vi "Send Plugin Command.vi"(6 "overwrite on timeout (T)":bool, 8 "error in (no error)":errorcluster, 9 "timeout in ms (0)":i32 format="%d ms", 10 "command":T1={"Command"=enum."Rx", "Parameters"={"arg1"=0, "arg2"=0}}, 11 "Plugin Interface in":refnum<class "Plugin Interface.lvclass">) -> (0 "error out":errorcluster, 3 "Plugin Interface out":refnum<class "Plugin Interface.lvclass">)   [LabVIEW 2020, in "DSF Core.lvlib" / "Plugin Interface.lvclass"]
uses:
  Plugin Interface.lvclass
  Interface.lvclass
  C:/Users/nitest/Desktop/Git/niveristand-data-sharing-framework-custom-device/Source/Core/Classes/Interface/Interface.lvclass
  C:/Users/nitest/Desktop/Git/niveristand-data-sharing-framework-custom-device/Source/Core/Classes/Interface/Plugin/Plugin Interface.lvclass
  Dispatcher/Command Timeout.vi
  DSF Core.lvlib
  Command.ctl
  Command Data.ctl
  Command Parameters.ctl
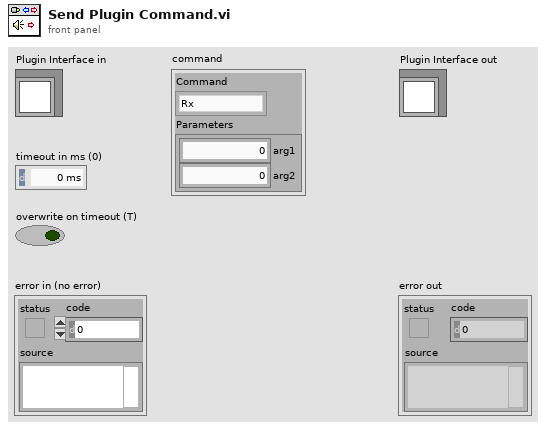
[diagram p1: front panel]
types:
  T1 = typedef "DSF Core.lvlib/Plugin Interface.lvclass/Command Data.ctl" = cluster{"Command":T2, "Parameters":T3}
  T2 = typedef "DSF Core.lvlib/Plugin Interface.lvclass/Command.ctl" = enum8{"Idle", "Start", "Set Inline Buffer", "Rx", "Tx", "Shutdown", "Error"}
  T3 = typedef "DSF Core.lvlib/Plugin Interface.lvclass/Command Parameters.ctl" = cluster{"arg1":u64, "arg2":u64}
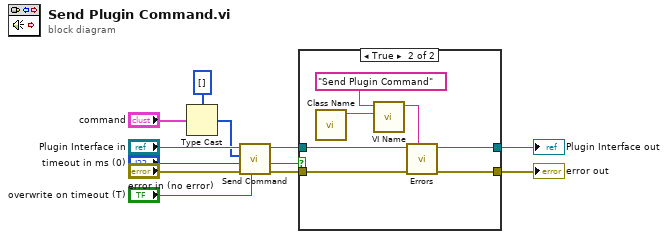
[diagram p0: block diagram]
diagram:
  n1 = Type Cast(type=u8[] [] ("element"), x="command") -> (*(type *) &x=w10:u8[])
  n2 = call "Send Command.vi"("overwrite on timeout (T)"="overwrite on timeout (T)", "error in (no error)"="error in (no error)", "timeout in ms (0)"="timeout in ms (0)", "command data"=w10, "Interface in"="Plugin Interface in") -> ("error out"=w5:errorcluster, "timed out?"=w4:bool, "Interface out"=w6:refnum<class "Plugin Interface.lvclass">)  [unwired: 3 in, 1 out]
  n3 = case shown="True" w4 {
    tunnel: w5 -> [w13 w20]
    tunnel: w6 -> [w14 w21]
    tunnel: [w14 w19] -> w3
    tunnel: [w13 w18] -> w2
    frame False {
    }
    frame True {
      n4 = call "Class Name.vi"() -> ("class name"=w17:string)  [unwired: 11 in]
      n5 = call "VI Name.vi"("class name (\"\")"=w17, "vi name"="Send Plugin Command" ("error source vi name")) -> ("full VI name"=w15:string)  [unwired: 9 in]
      n6 = call-poly "Errors.vi"("error source vi name"=w15, "error in (no error)"=w20, "Interface in"=w21) -> ("error out"=w18:errorcluster, "Interface out"=w19:refnum<class "Plugin Interface.lvclass">)  [unwired: 7 in]
    }
  }
  "error out" <- w2
  "Plugin Interface out" <- w3
